vi "NF WF1973_74 FUNC.vi"(6 "Read(F)":bool, 8 "error in (no error)":errorcluster caption="Error IN", 9 "Select Function(Sin)":i32(ring)=2 items=["DC", "Noise", "Sinusoid", "Square", "Pulse", "Ramp", "USine", "CSine", "CFCSine", "ACSine", "SSine", "MCSine", "ONPSine", "OFPSine", "CONSine", "COFSine", "Gaussian", "Lorents", "Haversine", "HSPulse", "TPulse", "Sinc", "ERise", "Efall", "Solstep", "Doscillation", "OSurge", "PSurge", "TOffset", "HSEPulse", "BRRamp", "USER"], 10 "Ch?(Ch1)":bool, 11 "VISAsession":refnum<visa-resource-name>) -> (0 "error out":errorcluster caption="Error OUT", 2 "Query Function":string, 3 "CopyVISAsession":refnum<visa-resource-name>)   [LabVIEW 2010]
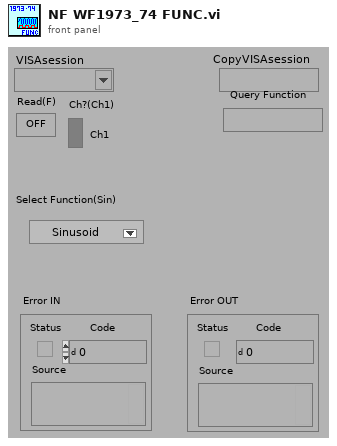
[diagram p1: front panel]
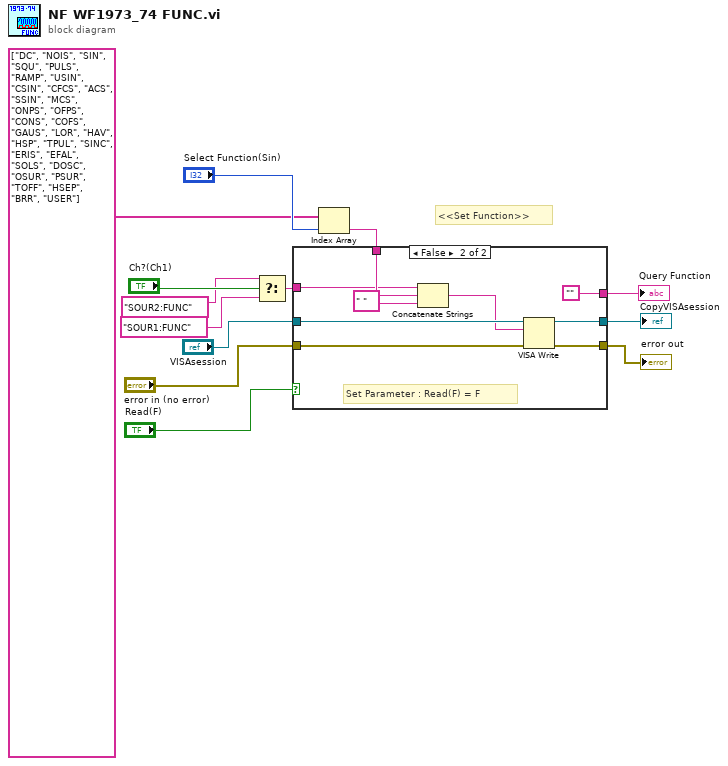
[diagram p0: block diagram]
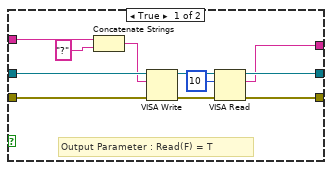
[diagram p2: hidden frame]
diagram:
  # "<<Set Function>>"
  n1 = Select(t="SOUR2:FUNC" ("文字列"), s="Ch?(Ch1)", f="SOUR1:FUNC" ("文字列")) -> (s? t:f=w4:string)
  n2 = Index Array(array=string[] ["DC", "NOIS", "SIN", "SQU", "PULS", "RAMP", "USIN", "CSIN", "CFCS", "ACS", "SSIN", "MCS", "ONPS", "OFPS", "CONS", "COFS", "GAUS", "LOR", "HAV", "HSP", "TPUL", "SINC", "ERIS", "EFAL", "SOLS", "DOSC", "OSUR", "PSUR", "TOFF", "HSEP", "BRR", "USER"], index="Select Function(Sin)") -> (element=w6:string)
  n3 = case shown="FALSE" "Read(F)" {
    tunnel: "VISAsession" -> [w24 w33]
    tunnel: [w21 w30] -> w12
    tunnel: [w20 w31] -> w11
    tunnel: "error in (no error)" -> [w19 w32]
    tunnel: w4 -> [w17 w25]
    tunnel: [w14 ""] -> w8
    tunnel: w6 -> [_ w27]
    frame True {
      # "Output Parameter : Read(F) = T"
      n4 = Concatenate Strings(w17, "?" ("形式文字列")) -> (w15:string)
      n5 = VISA Write(VISA resource name=w24, write buffer=w15, error in (no error)=w19) -> (VISA resource name out=w22:refnum<visa-resource-name>, error out=w23:errorcluster)  [unwired: 1 out]
      n6 = VISA Read(VISA resource name=w22, byte count=u32 10 ("バイトカウント（0）"), error in (no error)=w23) -> (VISA resource name out=w21:refnum<visa-resource-name>, read buffer=w14:string, error out=w20:errorcluster)  [unwired: 1 out]
    }
    frame False {
      # "Set Parameter : Read(F) = F"
      n7 = Concatenate Strings(w25, " ", w27) -> (w28:string)
      n8 = VISA Write(VISA resource name=w33, write buffer=w28, error in (no error)=w32) -> (VISA resource name out=w30:refnum<visa-resource-name>, error out=w31:errorcluster)  [unwired: 1 out]
    }
  }
  "error out" <- w11
  "CopyVISAsession" <- w12
  "Query Function" <- w8
